vi "SW_Plot_Thick_arc_line_IMAQdx.vi"(4 "Drawing Mode (Frame)":u32(ring) items=["Frame", "Fill"], 5 "End Angle (degrees)":dbl=70.0 format="%#_13g", 6 "Color":u32(colorbox), 7 "Start Angle (degrees)":dbl=110.0 format="%#_13g", 8 "Grow arc outside (T)":bool, 9 "Arc thickness, pix":u32=1, 10 "Bounding rectangle for outer segments, pix":T2, 11 "Picture in":T1) -> (3 "Picture out":T1)   [LabVIEW 2018, in "Tracker.lvlib"]
uses:
  <vilib>/vision/Image Controls.llb/IMAQ Image.ctl
  Tracker.lvlib
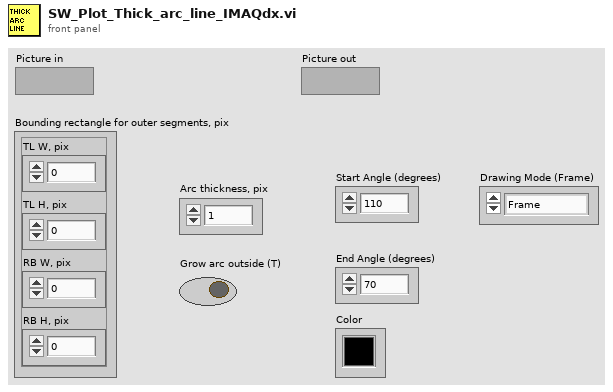
[diagram p1: front panel]
types:
  T1 = typedef "IMAQ Image.ctl" = refnum<image>
  T2 = cluster{"TL W, pix":i32, "TL H, pix":i32, "RB W, pix":i32, "RB H, pix":i32}
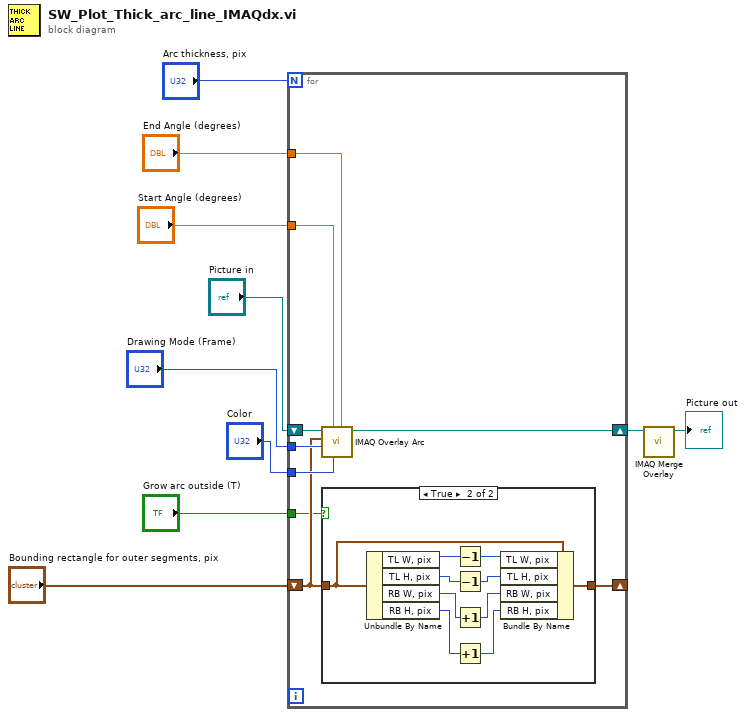
[diagram p0: block diagram]
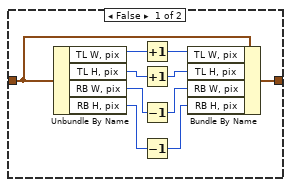
[diagram p2: hidden frame]
diagram:
  n1 = for {
    N: "Arc thickness, pix" -> [_]
    tunnel: "End Angle (degrees)" -> [w19]
    tunnel: "Color" -> [w18]
    tunnel: "Start Angle (degrees)" -> [w17]
    shift-right: [w15] -> w4
    shift-left: "Picture in" -> [w16]
    tunnel: "Drawing Mode (Frame)" -> [w14]
    shift-right: [w12] -> _
    shift-left: "Bounding rectangle for outer segments, pix" -> [w13]
    tunnel: "Grow arc outside (T)" -> [w11]
    n2 = call "IMAQ Overlay Arc"("End Angle (degrees)"=w19, "Color"=w18, "Start Angle (degrees)"=w17, "Drawing Mode (Frame)"=w14, "Bounding Rectangle"=w13, "Image"=w16) -> ("Image Out"=w15:T1)  [unwired: 4 in, 1 out]
    n3 = case shown="True" w11 {
      tunnel: w13 -> [w20 w30]
      tunnel: [w29 w39] -> w12
      frame False {
        n4 = Unbundle By Name(w20) -> ("TL W, pix"=w28:i32, "TL H, pix"=w26:i32, "RB W, pix"=w24:i32, "RB H, pix"=w22:i32)
        n5 = Increment(x=w28) -> (x+1=w27:i32)
        n6 = Increment(x=w26) -> (x+1=w25:i32)
        n7 = Decrement(x=w24) -> (x-1=w23:i32)
        n8 = Decrement(x=w22) -> (x-1=w21:i32)
        n9 = Bundle By Name(cluster=w20, "TL W, pix"=w27, "TL H, pix"=w25, "RB W, pix"=w23, "RB H, pix"=w21) -> (w29:T2)
      }
      frame True {
        n10 = Unbundle By Name(w30) -> ("TL W, pix"=w38:i32, "TL H, pix"=w36:i32, "RB W, pix"=w34:i32, "RB H, pix"=w32:i32)
        n11 = Decrement(x=w38) -> (x-1=w37:i32)
        n12 = Decrement(x=w36) -> (x-1=w35:i32)
        n13 = Increment(x=w34) -> (x+1=w33:i32)
        n14 = Increment(x=w32) -> (x+1=w31:i32)
        n15 = Bundle By Name(cluster=w30, "TL W, pix"=w37, "TL H, pix"=w35, "RB W, pix"=w33, "RB H, pix"=w31) -> (w39:T2)
      }
    }
  }
  n16 = call "IMAQ Merge Overlay"("Image Src"=w4) -> ("Image Dst Out"=→"Picture out":T1)  [unwired: 9 in, 1 out]
